vi "Arithmetic-Operations_(SubVI).vi"(10 "Numeric 2":dbl, 11 "Numeric":dbl) -> (1 "Numeric 3":dbl, 2 "Numeric 4":dbl, 3 "Numeric 6":dbl, 4 "Numeric 5":dbl)   [LabVIEW 2025]
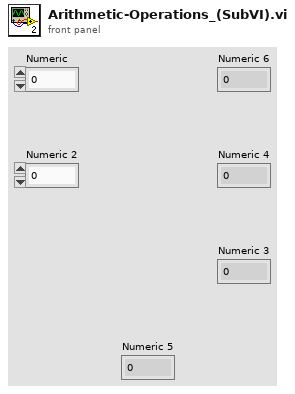
[diagram p1: front panel]
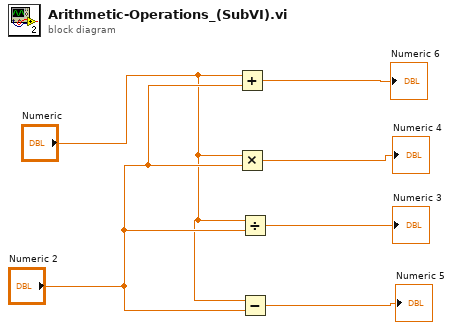
[diagram p0: block diagram]
diagram:
  n1 = Add(x="Numeric", y="Numeric 2") -> (x+y=→"Numeric 6":dbl)
  n2 = Multiply(x="Numeric", y="Numeric 2") -> (x*y=→"Numeric 4":dbl)
  n3 = Divide(x="Numeric", y="Numeric 2") -> (x/y=→"Numeric 3":dbl)
  n4 = Subtract(x="Numeric", y="Numeric 2") -> (x-y=→"Numeric 5":dbl)
